vi "MH_EnQError.vi"(8 "error in (no error)":errorcluster, 11 "Cmds_in":T1[](array[typedef])) -> (0 "error out":errorcluster, 3 "Cmds_out":T1[](array[typedef]))   [LabVIEW 2017]
uses:
  Types/MH_UIThread_Cmds.ctl
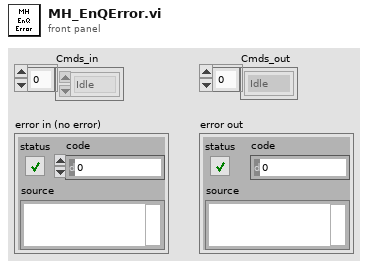
[diagram p1: front panel]
types:
  T1 = typedef "MH_UIThread_Cmds.ctl" = enum16{"Idle", "Init", "SetInpChan", "SetSyncDivider", "SetSyncTrg", "SetSyncOffset", "SetSyncDeadTime", "SetBinning", "SetHistoOffset", "SetHistoLen", "SetStopOvl", "SetBitShift", "SetHistoAcqTime", "GetRates", "GetAllRates", "StartMeas", "StopMeas", "AbortMeas", "GetResolution", "GetHistos", "GetAllHistos", "ReadFiFo", "WriteStatus", "Resize", "EnableControls", "DisableControls", "Error", "Exit"}
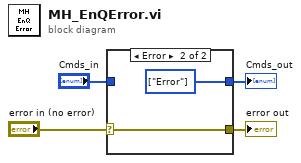
[diagram p0: block diagram]
diagram:
  n1 = case shown="Error" "error in (no error)" {
    selector: "error in (no error)" -> [_ w7]
    tunnel: [_ w7] -> w2
    tunnel: "Cmds_in" -> [w5 _]
    tunnel: [w5 w6] -> w4
    frame No Error {
    }
    frame Error {
      w6 = T1[] [enum."Error"] items=["Idle", "Init", "SetInpChan", "SetSyncDivider", "SetSyncTrg", "SetSyncOffset", "SetSyncDeadTime", "SetBinning", "SetHistoOffset", "SetHistoLen", "SetStopOvl", "SetBitShift", "SetHistoAcqTime", "GetRates", "GetAllRates", "StartMeas", "StopMeas", "AbortMeas", "GetResolution", "GetHistos", "GetAllHistos", "ReadFiFo", "WriteStatus", "Resize", "EnableControls", "DisableControls", "Error", "Exit"]
    }
  }
  "Cmds_out" <- w4
  "error out" <- w2
